vi "Process Menu Selection.vi"(8 "error in (no error)":errorcluster, 10 "Argument":string, 11 "Menu Ref":refnum<k9>) -> (0 "error out":errorcluster, 3 "State(s) to Enqueue":string)   [LabVIEW 2023, in "VI Properties Editor.lvlib"]
doc: "Processes a menu selection that occurred within the main window."
uses:
  VI Properties Editor.lvlib
  <vilib>/Utility/error.llb/Error Cluster From Error Code.vi
  <vilib>/ErrorRing/Error Ring.xnode
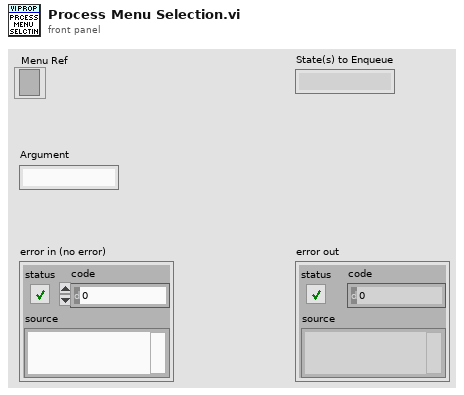
[diagram p1: front panel]
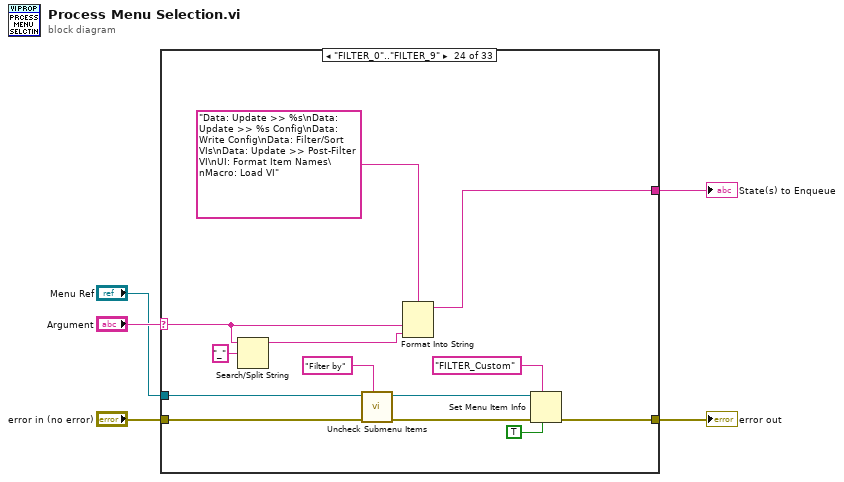
[diagram p0: block diagram]
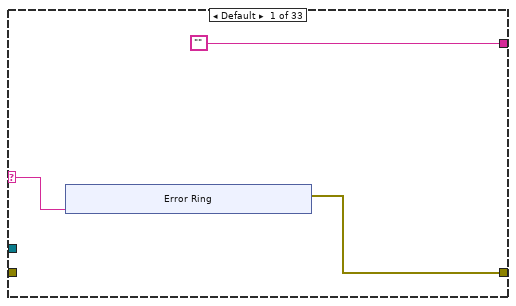
[diagram p2: hidden frame]
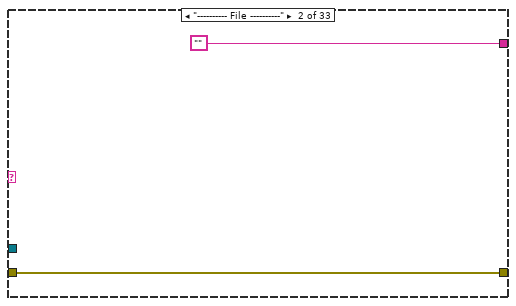
[diagram p3: hidden frame]
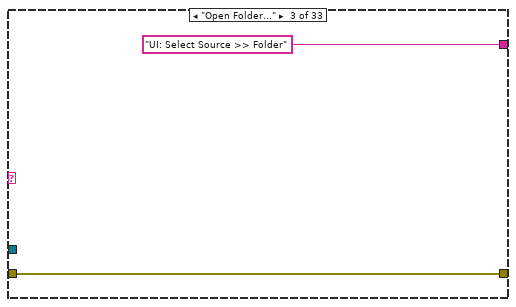
[diagram p4: hidden frame]
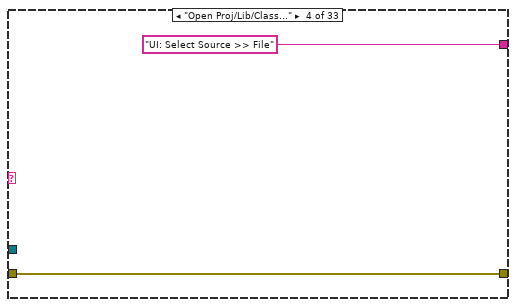
[diagram p5: hidden frame]
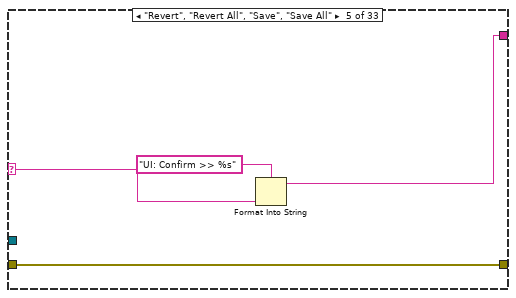
[diagram p6: hidden frame]
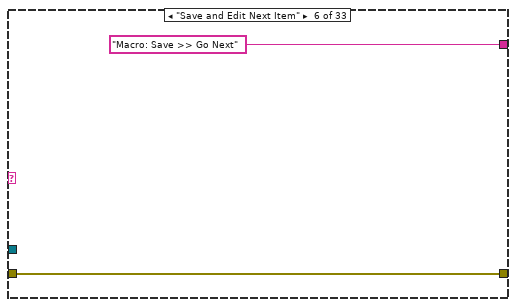
[diagram p7: hidden frame]
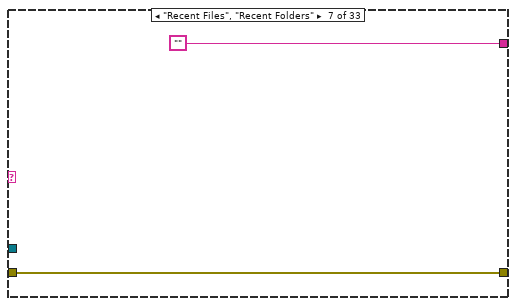
[diagram p8: hidden frame]
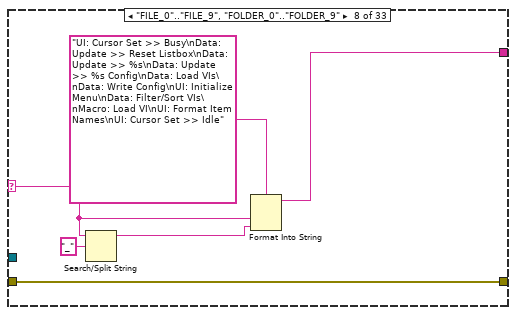
[diagram p9: hidden frame]
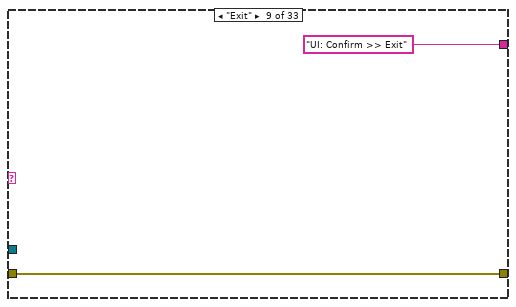
[diagram p10: hidden frame]
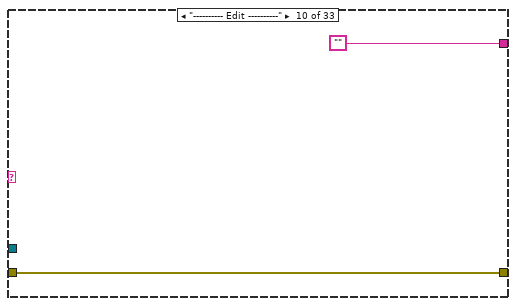
[diagram p11: hidden frame]
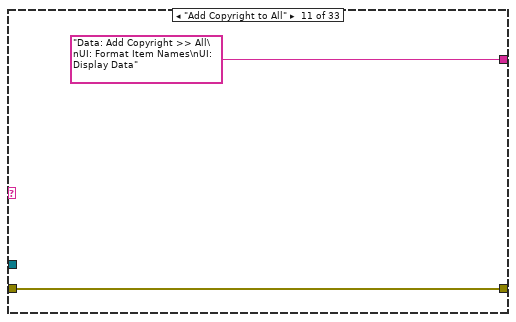
[diagram p12: hidden frame]
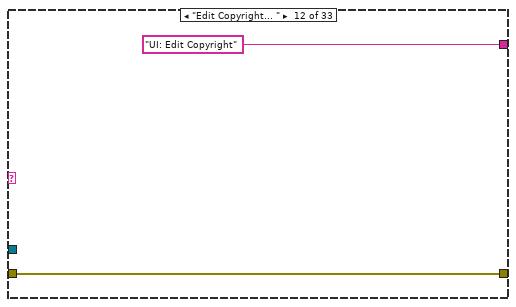
[diagram p13: hidden frame]
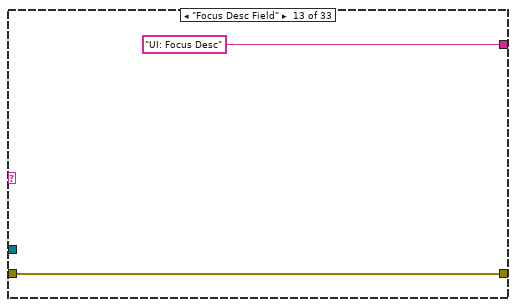
[diagram p14: hidden frame]
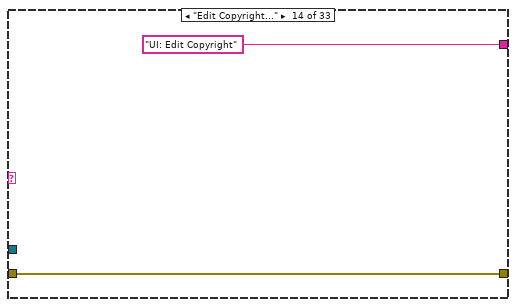
[diagram p15: hidden frame]
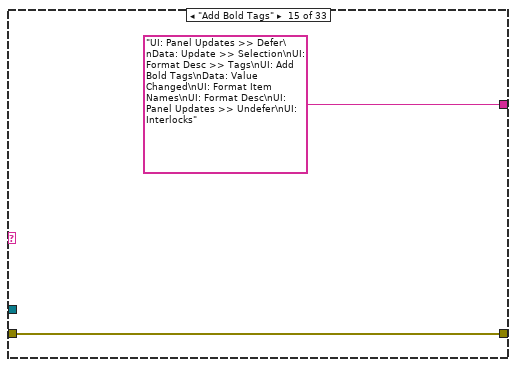
[diagram p16: hidden frame]
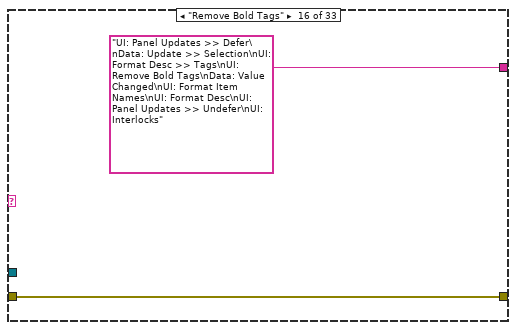
[diagram p17: hidden frame]
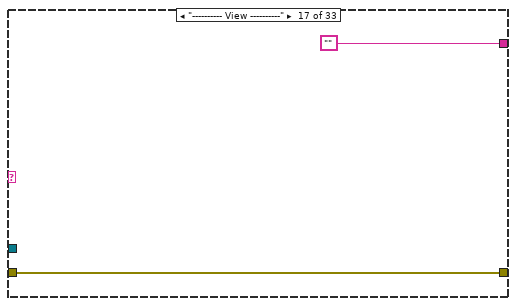
[diagram p18: hidden frame]
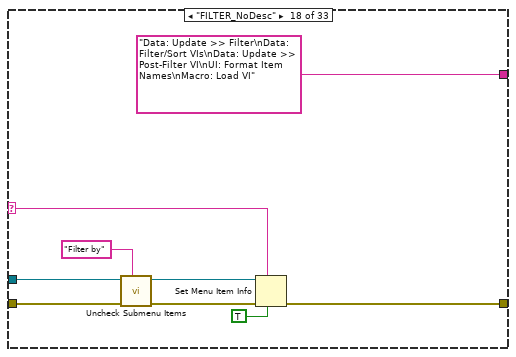
[diagram p19: hidden frame]
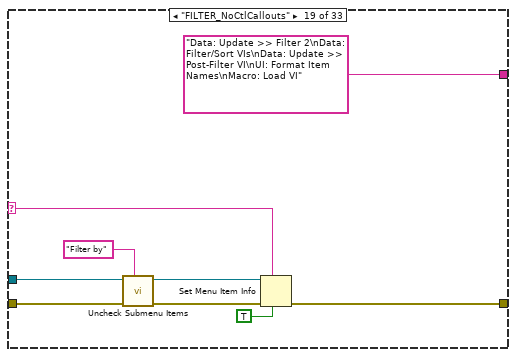
[diagram p20: hidden frame]
diagram:
  n1 = case shown="\"FILTER_0\"..\"FILTER_9\"" "Argument" {
    selector: "Argument" -> [w6 _ _ _ w23 _ _ w31 _ _ _ _ _ _ _ _ _ w59 w68 w77 _ w84 _ w105 w115 w119 w134 w143 _ w154 w168 w177 _]
    tunnel: ["" "" "UI: Select Source >> Folder" "UI: Select Source >> File" w22 "Macro: Save >> Go Next" "" w33 "UI: Confirm >> Exit" "" "Data: Add Copyright >> All\nUI: Format Item Names\nUI: Display Data" "UI: Edit Copyright" "UI: Focus Desc" "UI: Edit Copyright" "UI: Panel Updates >> Defer\nData: Update >> Selection\nUI: Format Desc >> Tags\nUI: Add Bold Tags\nData: Value Changed\nUI: Format Item Names\nUI: Format Desc\nUI: Panel Updates >> Undefer\nUI: Interlocks" "UI: Panel Updates >> Defer\nData: Update >> Selection\nUI: Format Desc >> Tags\nUI: Remove Bold Tags\nData: Value Changed\nUI: Format Item Names\nUI: Format Desc\nUI: Panel Updates >> Undefer\nUI: Interlocks" "" "Data: Update >> Filter\nData: Filter/Sort VIs\nData: Update >> Post-Filter VI\nUI: Format Item Names\nMacro: Load VI" "Data: Update >> Filter 2\nData: Filter/Sort VIs\nData: Update >> Post-Filter VI\nUI: Format Item Names\nMacro: Load VI" "Data: Update >> Clear Filter\nData: Filter/Sort VIs\nData: Update >> Post-Filter VI\nUI: Format Item Names\nMacro: Load VI" "UI: Add Custom Filter" "Data: Update >> Filter Config\nData: Write Config\nUI: Initialize Menu\nData: Filter/Sort VIs\nData: Update >> Post-Filter VI\nUI: Format Item Names\nMacro: Load VI" "" w107 "Data: Update >> Filter Data Source\nData: Filter/Sort VIs\nData: Update >> Post-Filter VI\nUI: Format Item Names\nMacro: Load VI" w118 "Data: Update >> Unsort\nData: Filter/Sort VIs\nData: Update >> Post-Filter VI\nUI: Format Item Names\nMacro: Load VI" "Data: Update >> Sort Order\nData: Filter/Sort VIs\nData: Update >> Post-Filter VI\nUI: Format Item Names\nMacro: Load VI" "" "Data: Update >> Abbr Names?\nUI: Format Item Names\nData: Write Config" w159 "Data: Update >> ShowCPCtlsOnly?\nData: Write Config\nData: Update >> All Ctls\nUI: Display Data" "UI: Edit Options"] -> w5
    tunnel: "Menu Ref" -> [_ _ _ _ _ _ _ _ _ _ _ _ _ _ _ _ _ w56 w65 w75 _ w90 _ w96 w116 w123 w135 w144 _ w155 w169 w178 _]
    tunnel: "error in (no error)" -> [_ w16 w18 w20 w25 w26 w28 w35 w37 w39 w40 w42 w44 w46 w48 w50 w53 w60 w69 w78 w81 w92 w94 w99 w110 w124 w133 w140 w147 w149 w164 w173 w179]
    tunnel: [w7 w16 w18 w20 w25 w26 w28 w35 w37 w39 w40 w42 w44 w46 w48 w50 w53 w58 w67 w72 w81 w87 w94 w98 w109 w127 w132 w139 w147 w148 w163 w172 w179] -> w4
    frame Default {
      n2 = xnode "Error Ring"("parameter 0"=w6) -> ("error out"=w7:errorcluster)
    }
    frame "---------- File ----------" {
    }
    frame "Open Folder..." {
    }
    frame "Open Proj/Lib/Class..." {
    }
    frame "Revert", "Revert All", "Save", "Save All" {
      n3 = Format Into String(format string="UI: Confirm >> %s", w23) -> (resulting string=w22:string)  [unwired: 2 in, 1 out]
    }
    frame "Save and Edit Next Item" {
    }
    frame "Recent Files", "Recent Folders" {
    }
    frame "FILE_0".."FILE_9", "FOLDER_0".."FOLDER_9" {
      n4 = Search/Split String(string=w31, search string/char (-)="_") -> (substring before match=w32:string)  [unwired: 1 in, 2 out]
      n5 = Format Into String(format string="UI: Cursor Set >> Busy\nData: Update >> Reset Listbox\nData: Update >> %s\nData: Update >> %s Config\nData: Load VIs\nData: Write Config\nUI: Initialize Menu\nData: Filter/Sort VIs\nMacro: Load VI\nUI: Format Item Names\nUI: Cursor Set >> Idle", w31, w32) -> (resulting string=w33:string)  [unwired: 2 in, 1 out]
    }
    frame "Exit" {
    }
    frame "---------- Edit ----------" {
    }
    frame "Add Copyright to All" {
    }
    frame "Edit Copyright... " {
    }
    frame "Focus Desc Field" {
    }
    frame "Edit Copyright..." {
    }
    frame "Add Bold Tags" {
    }
    frame "Remove Bold Tags" {
    }
    frame "---------- View ----------" {
    }
    frame "FILTER_NoDesc" {
      n6 = call "Uncheck Submenu Items.vi"("Item Tag"="Filter by", "error in (no error)"=w60, "Menu Ref"=w56) -> ("error out"=w57:errorcluster, "Menu Ref out"=w55:refnum<k9>)  [unwired: 7 in]
      n7 = Set Menu Item Info(6:TRUE ("checked"), 7:w59, 8:w57, 11:w55) -> (0:w58:errorcluster)  [unwired: 3 in, 1 out]
    }
    frame "FILTER_NoCtlCallouts" {
      n8 = call "Uncheck Submenu Items.vi"("Item Tag"="Filter by", "error in (no error)"=w69, "Menu Ref"=w65) -> ("error out"=w66:errorcluster, "Menu Ref out"=w64:refnum<k9>)  [unwired: 7 in]
      n9 = Set Menu Item Info(6:TRUE ("checked"), 7:w68, 8:w66, 11:w64) -> (0:w67:errorcluster)  [unwired: 3 in, 1 out]
    }
    frame "FILTER_Unfiltered" {
      n10 = call "Uncheck Submenu Items.vi"("Item Tag"="Filter by", "error in (no error)"=w78, "Menu Ref"=w75) -> ("error out"=w76:errorcluster, "Menu Ref out"=w74:refnum<k9>)  [unwired: 7 in]
      n11 = Set Menu Item Info(6:TRUE ("checked"), 7:w77, 8:w76, 11:w74) -> (0:w72:errorcluster)  [unwired: 3 in, 1 out]
    }
    frame "FILTER_Custom" {
    }
    frame "FILTER_Custom_Do" {
      n12 = call "Uncheck Submenu Items.vi"("Item Tag"="Filter by", "error in (no error)"=w92, "Menu Ref"=w90) -> ("error out"=w91:errorcluster, "Menu Ref out"=w89:refnum<k9>)  [unwired: 7 in]
      n13 = Search/Split String(string=w84, search string/char (-)="_Do") -> (substring before match=w83:string)  [unwired: 1 in, 2 out]
      n14 = Set Menu Item Info(6:TRUE ("checked"), 7:w83, 8:w91, 11:w89) -> (0:w87:errorcluster)  [unwired: 3 in, 1 out]
    }
    frame "Recent Filters" {
    }
    frame "FILTER_0".."FILTER_9" {
      n15 = Search/Split String(string=w105, search string/char (-)="_") -> (substring before match=w106:string)  [unwired: 1 in, 2 out]
      n16 = call "Uncheck Submenu Items.vi"("Item Tag"="Filter by", "error in (no error)"=w99, "Menu Ref"=w96) -> ("error out"=w103:errorcluster, "Menu Ref out"=w102:refnum<k9>)  [unwired: 7 in]
      n17 = Format Into String(format string="Data: Update >> %s\nData: Update >> %s Config\nData: Write Config\nData: Filter/Sort VIs\nData: Update >> Post-Filter VI\nUI: Format Item Names\nMacro: Load VI", w105, w106) -> (resulting string=w107:string)  [unwired: 2 in, 1 out]
      n18 = Set Menu Item Info(6:TRUE ("checked"), 7:"FILTER_Custom" ("item tag"), 8:w103, 11:w102) -> (0:w98:errorcluster)  [unwired: 3 in, 1 out]
    }
    frame "FILTER_DataSource" {
      n19 = Get Menu Item Info(7:w115, 8:w110, 11:w116) -> (0:w114:errorcluster, 3:w113:refnum<k9>, 4:w112:bool)  [unwired: 4 out]
      n20 = Not(x=w112) -> (.not. x?=w111:bool)
      n21 = Set Menu Item Info(6:w111, 7:w115, 8:w114, 11:w113) -> (0:w109:errorcluster)  [unwired: 3 in, 1 out]
    }
    frame "SORT_0".."SORT_99" {
      n22 = call "Uncheck Submenu Items.vi"("Item Tag"="Sort by" ("item tag"), "error in (no error)"=w124, "Menu Ref"=w123) -> ("error out"=w121:errorcluster, "Menu Ref out"=w122:refnum<k9>)  [unwired: 7 in]
      n23 = Set Menu Item Info(6:TRUE ("checked"), 7:w119, 8:w121, 11:w122) -> (0:w127:errorcluster)  [unwired: 3 in, 1 out]
      n24 = Format Into String(format string="Data: Update >> %s\nData: Filter/Sort VIs\nData: Update >> Post-Filter VI\nUI: Format Item Names\nMacro: Load VI", w119) -> (resulting string=w118:string)  [unwired: 2 in, 1 out]
    }
    frame "SORT_Unsorted" {
      n25 = call "Uncheck Submenu Items.vi"("Item Tag"="Sort by" ("item tag"), "error in (no error)"=w133, "Menu Ref"=w135) -> ("error out"=w128:errorcluster, "Menu Ref out"=w129:refnum<k9>)  [unwired: 7 in]
      n26 = Set Menu Item Info(6:TRUE ("checked"), 7:w134, 8:w128, 11:w129) -> (0:w132:errorcluster)  [unwired: 3 in, 1 out]
    }
    frame "SORT_Order" {
      n27 = Get Menu Item Info(7:w143, 8:w140, 11:w144) -> (0:w142:errorcluster, 3:w141:refnum<k9>, 4:w138:bool)  [unwired: 4 out]
      n28 = Not(x=w138) -> (.not. x?=w137:bool)
      n29 = Set Menu Item Info(6:w137, 7:w143, 8:w142, 11:w141) -> (0:w139:errorcluster)  [unwired: 3 in, 1 out]
    }
    frame "---------- Options ----------" {
    }
    frame "Abbr if Class in Lib" {
      n30 = Get Menu Item Info(7:w154, 8:w149, 11:w155) -> (0:w153:errorcluster, 3:w152:refnum<k9>, 4:w151:bool)  [unwired: 4 out]
      n31 = Not(x=w151) -> (.not. x?=w150:bool)
      n32 = Set Menu Item Info(6:w150, 7:w154, 8:w153, 11:w152) -> (0:w148:errorcluster)  [unwired: 3 in, 1 out]
    }
    frame "Format Bold Text" {
      n33 = Get Menu Item Info(7:w168, 8:w164, 11:w169) -> (0:w167:errorcluster, 3:w166:refnum<k9>, 4:w165:bool)  [unwired: 4 out]
      n34 = Not(x=w165) -> (.not. x?=w162:bool)
      n35 = Set Menu Item Info(6:w162, 7:w168, 8:w167, 11:w166) -> (0:w163:errorcluster)  [unwired: 3 in, 1 out]
      n36 = Select(t="UI: Format Desc", s=w162, f="UI: Format Desc >> Tags") -> (s? t:f=w157:string)
      n37 = Format Into String(format string="Data: Update >> Format Bold?\nData: Write Config\nUI: Display Data\n%s", w157) -> (resulting string=w159:string)  [unwired: 2 in, 1 out]
    }
    frame "Only Show ConPane Ctls" {
      n38 = Get Menu Item Info(7:w177, 8:w173, 11:w178) -> (0:w176:errorcluster, 3:w175:refnum<k9>, 4:w174:bool)  [unwired: 4 out]
      n39 = Not(x=w174) -> (.not. x?=w171:bool)
      n40 = Set Menu Item Info(6:w171, 7:w177, 8:w176, 11:w175) -> (0:w172:errorcluster)  [unwired: 3 in, 1 out]
    }
    frame "All Options..." {
    }
  }
  "error out" <- w4
  "State(s) to Enqueue" <- w5
